vi "AWGSwitchtoApp.vi"(2 "error in (no error)":errorcluster, 3 "Switch to App":u8(ring) items=["Simple AFG", "Serial Pattern Generator (SPG)"], 4 "VISA resource name":refnum<visa-resource-name>) -> (0 "error out":errorcluster, 1 "VISA resource name out":refnum<visa-resource-name>)   [LabVIEW 2020, in "Active Technologies AWG3000.lvlib"]
uses:
  Active Technologies AWG3000.lvlib
panel:
  # "Note: Digital Serial Pattern Generator  (SPG) is only available for  the AWG4000 serie with an active license."
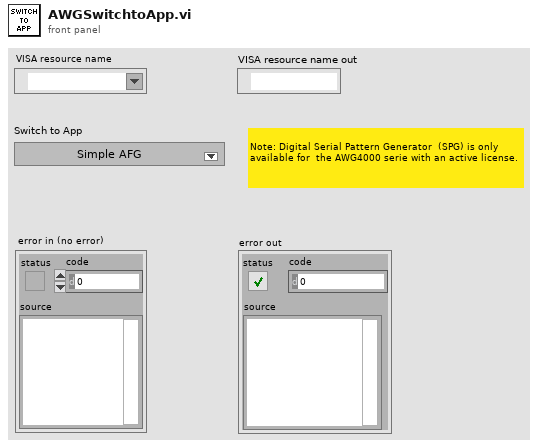
[diagram p1: front panel]
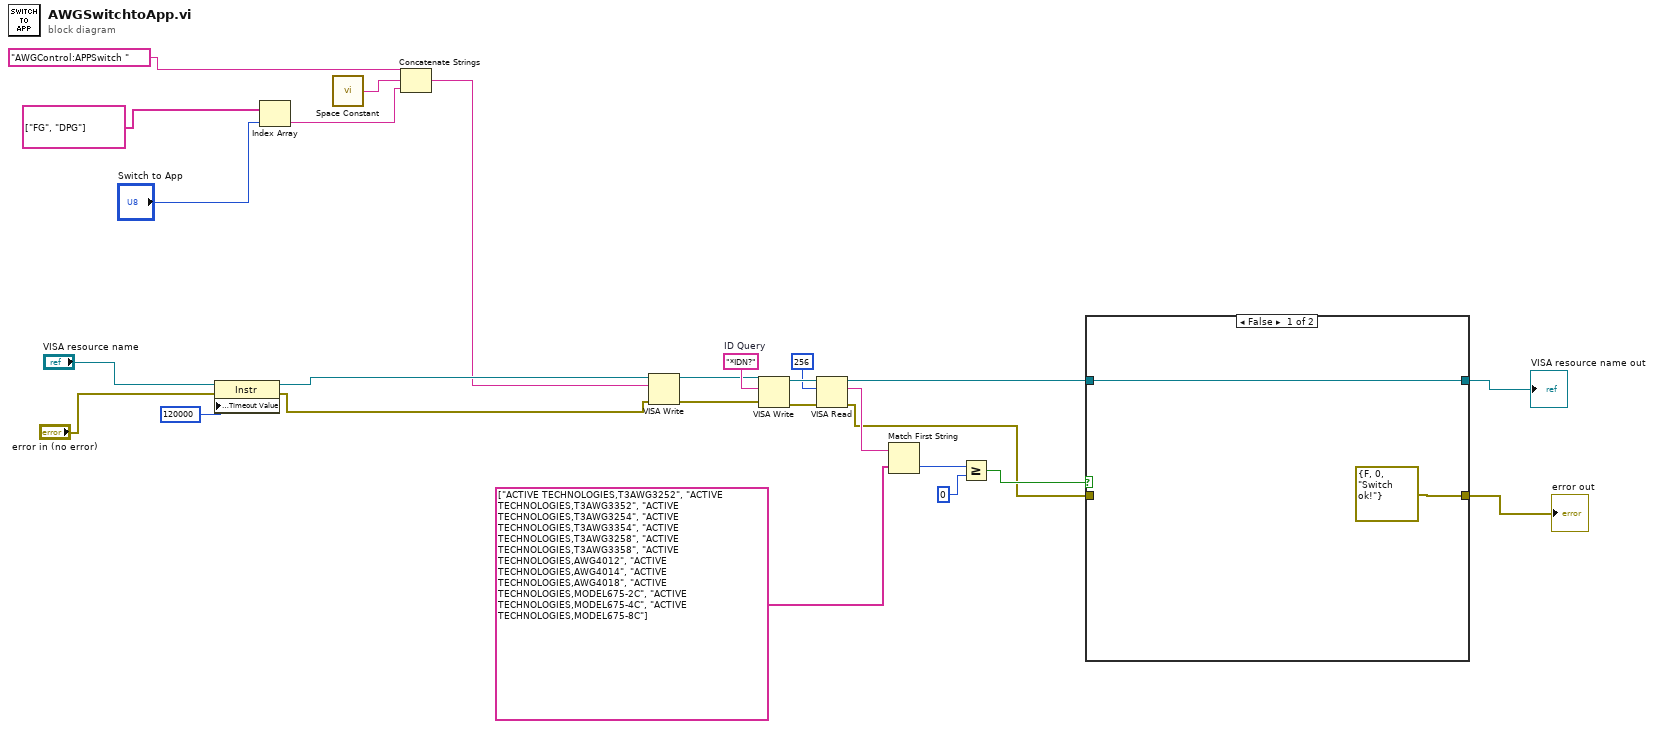
[diagram p0: block diagram]
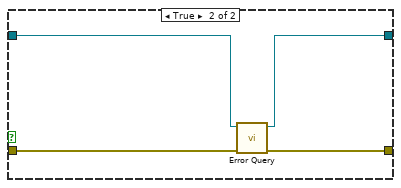
[diagram p2: hidden frame]
diagram:
  w19 = "*IDN?"  # ID Query
  n1 = property class="Instr"(reference="VISA resource name", error in="error in (no error)", "General Settings:Timeout Value"=u32 120000) -> (reference out=w23:refnum<visa-resource-name>, error out=w24:errorcluster)
  n2 = Index Array(array=string[] ["FG", "DPG"] ("reversed array"), index="Switch to App") -> (element=w5:string)
  n3 = call <vilib>:"Space Constant.vi"() -> ("String"=w4:string)
  n4 = Concatenate Strings("AWGControl:APPSwitch " ("write buffer"), w4, w5) -> (w2:string)
  n5 = VISA Write(VISA resource name=w23, write buffer=w2, error in (no error)=w24) -> (VISA resource name out=w9:refnum<visa-resource-name>, error out=w8:errorcluster)  [unwired: 1 out]
  n6 = VISA Write(VISA resource name=w9, write buffer=w19, error in (no error)=w8) -> (VISA resource name out=w22:refnum<visa-resource-name>, error out=w21:errorcluster)  [unwired: 1 out]
  n7 = VISA Read(VISA resource name=w22, byte count=u32 256, error in (no error)=w21) -> (VISA resource name out=w14:refnum<visa-resource-name>, read buffer=w18:string, error out=w13:errorcluster)  [unwired: 1 out]
  n8 = Match First String(2:string[] ["ACTIVE TECHNOLOGIES,T3AWG3252", "ACTIVE TECHNOLOGIES,T3AWG3352", "ACTIVE TECHNOLOGIES,T3AWG3254", "ACTIVE TECHNOLOGIES,T3AWG3354", "ACTIVE TECHNOLOGIES,T3AWG3258", "ACTIVE TECHNOLOGIES,T3AWG3358", "ACTIVE TECHNOLOGIES,AWG4012", "ACTIVE TECHNOLOGIES,AWG4014", "ACTIVE TECHNOLOGIES,AWG4018", "ACTIVE TECHNOLOGIES,MODEL675-2C", "ACTIVE TECHNOLOGIES,MODEL675-4C", "ACTIVE TECHNOLOGIES,MODEL675-8C"] ("reversed array"), 3:w18) -> (0:w17:i32)  [unwired: 1 out]
  n9 = Greater Or Equal?(x=w17, y=0) -> (x >= y?=w15:bool)
  n10 = case shown="False" w15 {
    tunnel: w14 -> [w28 w32]
    tunnel: w13 -> [_ w31]
    tunnel: [w28 w30] -> w12
    tunnel: [errorcluster {"status"=FALSE, "code"=0, "source"="Switch ok!"} ("error out") w29] -> w11
    frame False {
    }
    frame True {
      n11 = call "Error Query.vi"("error in (no error)"=w31, "VISA resource name"=w32) -> ("error out"=w29:errorcluster, "VISA resource name out"=w30:refnum<visa-resource-name>)  [unwired: 6 in, 2 out]
    }
  }
  "VISA resource name out" <- w12
  "error out" <- w11
